vi "Memory Benchmark.vi"(5 "Show Cache Lines (F)":bool, 7 "Show Peak Bandwidth (F)":bool, 9 "Transfers (500)":i32=500, 10 "End Size":u64=50000000 format="%.0pB", 11 "Start Size":u64=1000 format="%.0pB") -> (3 "Memory Bandwidth":cluster{"X":dbl[], "Y":dbl[]}[](graph) caption="Memory Bandwidth Plot")   [LabVIEW 2016]
uses:
  Source/Library/Classes/Pointer/Memory.Pointer.lvclass/Memory.Pointer.ctl
  Source/Library/Classes/Pointer/Methods/Memory.Pointer.Copy.Unsafe.vi
  Source/Library/Classes/Pointer/Accessors/Get Address.vi
  Source/Library/Classes/Pointer/Accessors/Set Address.vi
  Source/Library/Classes/Pointer/Accessors/Set Size.vi
  Source/Library/Classes/Pointer.Internal/Memory.Pointer.Internal.lvclass
  C:/Users/Ryan/Documents/Git/Sourcetree/LabVIEW-Memory-Manager/Source/Library/Classes/Pointer/Memory.Pointer.lvclass
  Source/Library/Classes/Pointer/Memory.Pointer.lvclass
panel:
  out "Peak Throughput":dbl format="%.3pB/s"
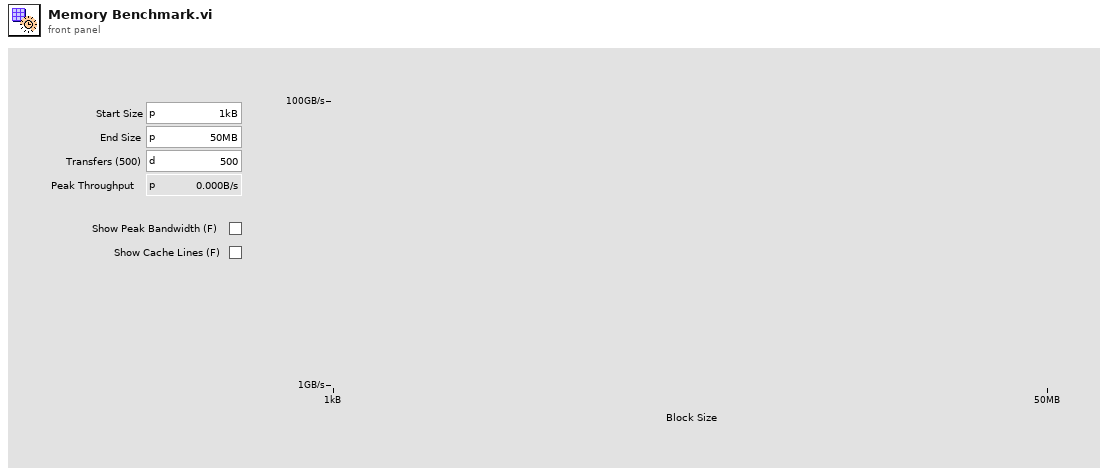
[diagram p1: front panel]
types:
  T1 = typedef "LVAnnotationListTypeDef.ctl" = cluster{"Name":string, "Color":u32, "Style":u8, "Point Style":u8, "Name Visible":bool, "Allow Drag":bool, "Annotation Mode":u32, "Plot":i32, "Index":i32, "Position":cluster{"X":dbl, "Y":dbl}, "X Scale":u32, "Y Scale":u32, "Show Arrow":bool, "Lock Name":bool, "Plot Area":i32, "Label Offset":cluster{"X":dbl, "Y":dbl}}[]
  T2 = cluster{"Name":string, "Color":u32, "Style":u8, "Point Style":u8, "Name Visible":bool, "Allow Drag":bool, "Annotation Mode":u32, "Plot":i32, "Index":i32, "Position":cluster{"X":dbl, "Y":dbl}, "X Scale":u32, "Y Scale":u32, "Show Arrow":bool, "Lock Name":bool, "Plot Area":i32, "Label Offset":cluster{"X":dbl, "Y":dbl}}
  T3 = cluster{"Name":string, "Color":u32, "Style":u8, "Point Style":u8, "Name Visible":bool, "Allow Drag":bool, "Annotation Mode":u32, "Plot":i32, "Index":i32, "Position":cluster{"X":dbl, "Y":dbl}, "X Scale":u32, "Y Scale":u32, "Show Arrow":bool, "Lock Name":bool, "Plot Area":i32, "Label Offset":cluster{"X":dbl, "Y":dbl}}[]
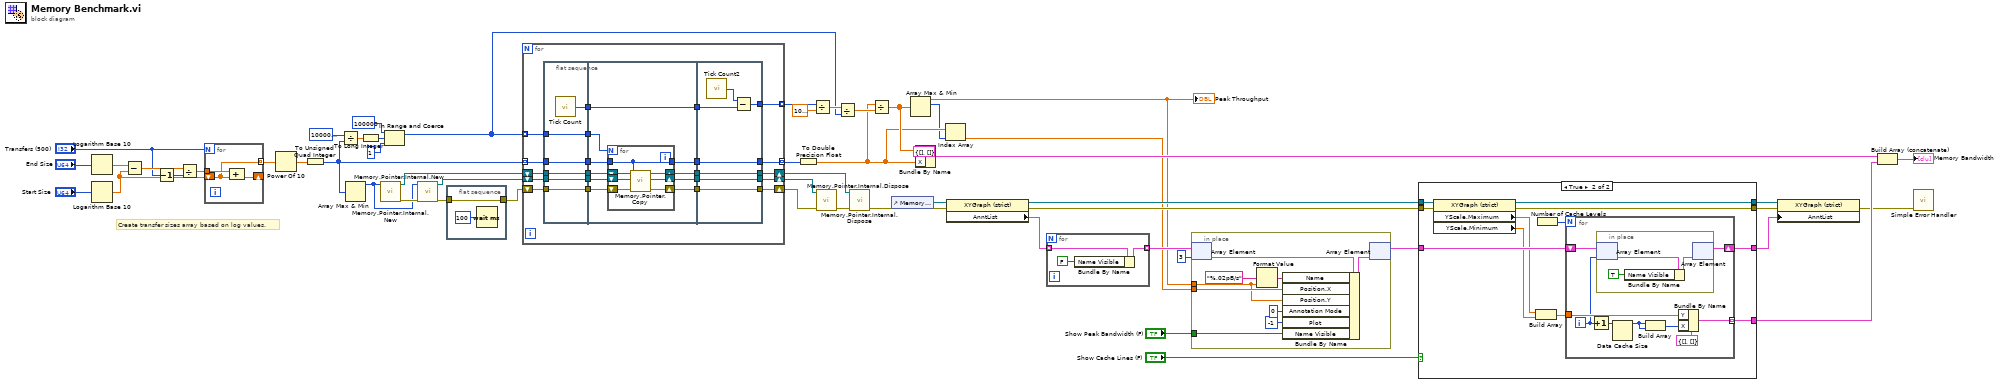
[diagram p0: block diagram]
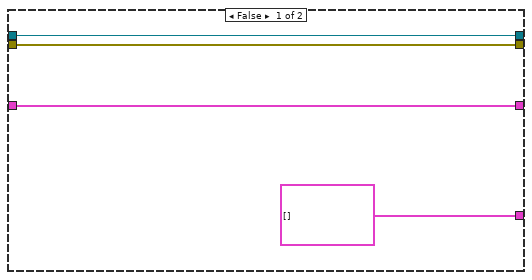
[diagram p2: hidden frame]
diagram:
  # "Create transfer sizes array based on log values."
  n1 = Logarithm Base 10(1:"End Size") -> (0:w53:dbl)
  n2 = Logarithm Base 10(1:"Start Size") -> (0:w50:dbl)
  n3 = Subtract(x=w53, y=w50) -> (x-y=w52:dbl)
  n4 = Decrement(x="Transfers (500)") -> (x-1=w48:i32)
  n5 = Divide(x=w52, y=w48) -> (x/y=w51:dbl)
  n6 = for {
    N: "Transfers (500)" -> [_]
    tunnel: w51 -> [w58]
    shift-right: [w57] -> _
    shift-left: w50 -> [w56]
    tunnel: [w56] -> w47 mode=indexing
    n7 = Compound Arithmetic op=ADD(w58, w56) -> (w57:dbl)
  }
  n8 = Power Of 10(x=w47) -> (10^x=w46:dbl[])
  n9 = To Unsigned Quad Integer(1:w46) -> (0:w40:u64[])
  n10 = Divide(x=u64 100000000, y=w40) -> (x/y=w39:dbl[])
  n11 = Array Max & Min(array=w40) -> (max value=w3:u64)  [unwired: 3 out]
  n12 = To Long Integer(number=w39) -> (32bit integer=w38:i32[])
  n13 = call "Memory.Pointer.Internal.New.vi"("size"=w3) -> ("error out"=w34:errorcluster, "pointer"=w24:refnum<class "Memory.Pointer.Internal.lvclass">)  [unwired: 9 in]
  n14 = In Range and Coerce(upper limit=100000, x=w38, lower limit=1) -> (coerced(x)=w17:i32[])  [unwired: 1 out]
  n15 = call "Memory.Pointer.Internal.New.vi"("error in (no error)"=w34, "size"=w3) -> ("error out"=w23:errorcluster, "pointer"=w35:refnum<class "Memory.Pointer.Internal.lvclass">)  [unwired: 8 in]
  n16 = flat-sequence {
    tunnel: w23 -> [w60]
    tunnel: [w60] -> w22
    frame #0 {
      n17 = Wait (ms)(milliseconds to wait=u32 100) -> ()  [unwired: 1 out]
    }
  }
  n18 = for {
    shift-right: [w65] -> w32
    shift-left: w35 -> [w69]
    shift-right: [w64] -> w30
    shift-left: w24 -> [w68]
    shift-right: [w66] -> w33
    shift-left: w22 -> [w67]
    tunnel: [w63] -> w28 mode=indexing
    tunnel: w40 -> [w62] mode=indexing
    tunnel: [w61] -> w25 mode=indexing
    tunnel: w17 -> [w70] mode=indexing
    n19 = flat-sequence {
      tunnel: [w87] -> w81
      tunnel: [w86] -> w80
      tunnel: [w85] -> w79
      tunnel: [w84] -> w78
      tunnel: [w83] -> w77
      tunnel: [w82] -> w76
      tunnel: w68 -> [w87]
      tunnel: w69 -> [w86]
      tunnel: w67 -> [w85]
      tunnel: w62 -> [w84]
      tunnel: w70 -> [w83]
      tunnel: w81 -> [w97]
      tunnel: w80 -> [w88]
      tunnel: w79 -> [w96]
      tunnel: w78 -> [w95]
      tunnel: w77 -> [w91]
      tunnel: w76 -> [w90]
      tunnel: [w90] -> w75
      tunnel: [w94] -> w74
      tunnel: [w93] -> w73
      tunnel: [w92] -> w72
      tunnel: [w89] -> w71
      tunnel: w75 -> [w110]
      tunnel: w74 -> [w109]
      tunnel: w73 -> [w108]
      tunnel: w72 -> [w107]
      tunnel: w71 -> [w106]
      tunnel: [w109] -> w66
      tunnel: [w108] -> w64
      tunnel: [w107] -> w65
      tunnel: [w106] -> w61
      tunnel: [w105] -> w63
      frame #0 {
        n20 = call "Tick Count"() -> ("Tick Count(uSec)"=w82:u32)
      }
      frame #1 {
        n21 = for {
          N: w91 -> [_]
          shift-right: [w101] -> w94
          shift-left: w96 -> [w102]
          shift-right: [w100] -> w93
          shift-left: w97 -> [w104]
          shift-right: [w99] -> w92
          shift-left: w88 -> [w103]
          tunnel: w95 -> [w98]
          tunnel: [w98] -> w89
          n22 = call-poly "Memory.Pointer.Copy.vi"("error in (no error)"=w102, "bytes to copy"=w98, "dst pointer in"=w103, "src pointer in"=w104) -> ("error out"=w101:errorcluster, "dst pointer out"=w99:refnum<class "Memory.Pointer.Internal.lvclass">, "src pointer out"=w100:refnum<class "Memory.Pointer.Internal.lvclass">)  [unwired: 4 in, 1 out]
        }
      }
      frame #2 {
        n23 = call "Tick Count2"() -> ("Tick Count(uSec)"=w111:u32)
        n24 = Subtract(x=w111, y=w110) -> (x-y=w105:u32)
      }
    }
  }
  n25 = To Double Precision Float(number=w25) -> (double precision float=w21:dbl[])
  n26 = Divide(x=w28, y=1000000.0) -> (x/y=w27:dbl[])
  n27 = call "Memory.Pointer.Internal.Dispose.vi"("error in (no error)"=w33, "pointer"=w32) -> ("error out"=w31:errorcluster)  [unwired: 9 in]
  n28 = Divide(x=w27, y=w17) -> (x/y=w26:dbl[])
  n29 = call "Memory.Pointer.Internal.Dispose.vi"("error in (no error)"=w31, "pointer"=w30) -> ("error out"=w7:errorcluster)  [unwired: 9 in]
  n30 = Divide(x=w21, y=w26) -> (x/y=w45:dbl[])
  n31 = control-ref of="Memory Bandwidth"() -> (w15:refnum<vi>)
  n32 = Array Max & Min(array=w45) -> (max value=w9:dbl, max index (indices)=w19:i32)  [unwired: 2 out]
  "Peak Throughput" <- w9
  n33 = Bundle By Name(cluster=cluster{"X":dbl[], "Y":dbl[]} {"X"=[], "Y"=[]}, "Y"=w45, "X"=w21) -> (w43:cluster{"X":dbl[], "Y":dbl[]})
  n34 = Index Array(array=w21, index=w19) -> (element=w8:dbl)
  n35 = property class="XYGraph (strict)"(reference=w15, error in=w7) -> (reference out=w10:refnum<vi>, error out=w11:errorcluster, "AnntList"=w14:T1)
  n36 = for {
    tunnel: w14 -> [w113] mode=indexing
    tunnel: [w112] -> w12 mode=indexing
    n37 = Bundle By Name(cluster=w113, "Name Visible"=FALSE) -> (w112:T2)
  }
  n38 = in-place {
    in-place-border: w9 -> [w115]
    in-place-border: w8 -> [w119]
    in-place-border: "Show Peak Bandwidth (F)" -> [w116]
    n39 = in-place-array #1(w12, 3) -> (w123:T2)
    n40 = Format Value(format string="%.02pB/s", value (0)=w115) -> (output string=w121:string)  [unwired: 1 in]
    n41 = Bundle By Name(cluster=w123, "Name"=w121, "Position.X"=w119, "Position.Y"=w115, "Annotation Mode"=u32 0, "Plot"=-1, "Name Visible"=w116) -> (w120:T2)
    n42 = in-place-array #1(w120) -> (w16:T3)  [unwired: 1 out]
  }
  n43 = case shown="True" "Show Cache Lines (F)" {
    tunnel: [cluster{"X":dbl[], "Y":dbl[]}[] [] w136] -> w2
    tunnel: w10 -> [w124 w135]
    tunnel: w16 -> [w125 w134]
    tunnel: w11 -> [w126 w133]
    tunnel: [w126 w130] -> w6
    tunnel: [w124 w129] -> w5
    tunnel: [w125 w128] -> w4
    frame False {
    }
    frame True {
      n44 = property class="XYGraph (strict)"(reference=w135, error in=w133) -> (reference out=w129:refnum<vi>, error out=w130:errorcluster, "YScale.Maximum"=w132:dbl, "YScale.Minimum"=w131:dbl)
      n45 = Build Array(w132, w131) -> (w137:dbl[])
      n46 = Number of Cache Levels() -> (w138:i32)
      n47 = for {
        N: w138 -> [_]
        tunnel: w137 -> [w143]
        tunnel: [w142] -> w136 mode=indexing
        shift-right: [w140] -> w128
        shift-left: w134 -> [w141]
        i -> [w139]
        n48 = Increment(x=w139) -> (x+1=w147:i32)
        n49 = in-place {
          n50 = in-place-array #2(w141, w139) -> (w150:T2)
          n51 = Bundle By Name(cluster=w150, "Name Visible"=TRUE) -> (w149:T2)
          n52 = in-place-array #2(w149) -> (w140:T3)  [unwired: 1 out]
        }
        n53 = Data Cache Size(0:w147) -> (4:w145:i32)  [unwired: 1 out]
        n54 = Build Array(w145, w145) -> (w144:i32[])
        n55 = Bundle By Name(cluster=cluster{"X":dbl[], "Y":dbl[]} {"X"=[], "Y"=[]}, "Y"=w143, "X"=w144) -> (w142:cluster{"X":dbl[], "Y":dbl[]})
      }
    }
  }
  n56 = property class="XYGraph (strict)"(reference=w5, error in=w6, "AnntList"=w4) -> (error out=w1:errorcluster)  [unwired: 1 out]
  n57 = Build Array (concatenate)(w43, w2) -> (→"Memory Bandwidth":cluster{"X":dbl[], "Y":dbl[]}[])
  n58 = call <vilib>:"Simple Error Handler.vi"("error in (no error)"=w1) -> ()  [unwired: 4 in, 5 out]
